vi "Areotech set reset.vi"(8 "error in (no error)":errorcluster, 10 "Parsed CMD":T1, 11 "AerotechStage in":refnum<class "AerotechStage.lvclass">) -> (0 "error out":errorcluster, 2 "new commands":string, 3 "AerotechStage out":refnum<class "AerotechStage.lvclass">)   [LabVIEW 2020, in "AerotechStage.lvclass"]
uses:
  AerotechStage.lvclass
  parsed device cmd.ctl
  OnOffTypeDef.ctl
  AerotechStage.lvclass/AerotechStage.ctl
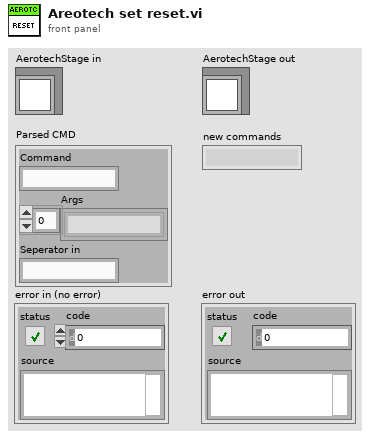
[diagram p1: front panel]
types:
  T1 = typedef "parsed device cmd.ctl" = cluster{"Command":string, "Args":string[], "Seperator in":string}
  T2 = typedef "OnOffTypeDef.ctl" = enum16{"off", "on"}
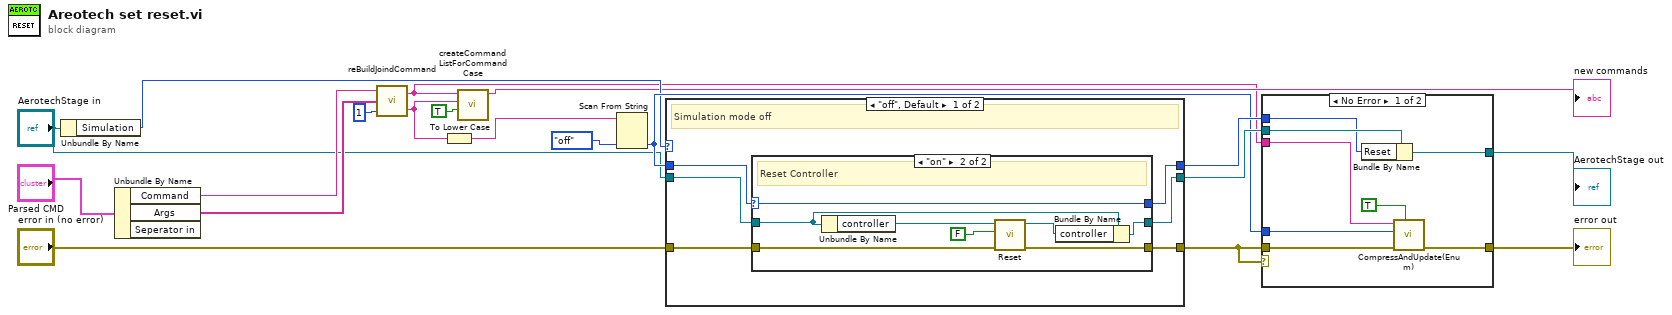
[diagram p0: block diagram]
diagram:
  n1 = Unbundle By Name("AerotechStage in") -> ("Simulation"=w7:T2)
  n2 = Unbundle By Name("Parsed CMD") -> ("Command"=w18:string, "Args"=w19:string[])  [unwired: 1 out]
  n3 = call "reBuildJoindCommand.vi"("number of group elements (0)"=1, "Args"=w19, "Command 2"=w18) -> ("Arg"=w9:string, "Command"=w3:string)
  n4 = To Lower Case(string=w9) -> (all lower case string=w8:string)
  n5 = call "createCommandListForCommandCase.vi"("immediate Check (only once)"=TRUE, "setvalue"=w9, "command"=w3) -> ("new commands"=→"new commands":string)  [unwired: 8 in]
  n6 = Scan From String(input string=w8, default 1=OnOffTypeDef."off" ("Settings.Enable.Axis 1")) -> (output 1=w11:T2)  [unwired: 3 in, 3 out]
  n7 = case shown="\"off\", Default" w7 {
    tunnel: "AerotechStage in" -> [w25 w39]
    tunnel: "error in (no error)" -> [w23 w38]
    tunnel: [w22 w38] -> w16
    tunnel: [w24 w39] -> w13
    tunnel: w11 -> [w21 w37]
    tunnel: [w20 w37] -> w15
    frame "off", Default {
      # "Simulation mode off"
      n8 = case shown="\"on\"" w21 {
        selector: w21 -> [w26 w29]
        tunnel: w25 -> [w27 w34]
        tunnel: [w27 w33] -> w24
        tunnel: w23 -> [w28 w36]
        tunnel: [w28 w35] -> w22
        tunnel: [w26 w29] -> w20
        frame "off", Default {
        }
        frame "on" {
          # "Reset Controller"
          n9 = Unbundle By Name(w34) -> ("controller"=w32:refnum<k24>)
          n10 = call "Reset.vi"("error in (no error)"=w36, "restart programs? (false)"=FALSE, "controller in"=w32) -> ("error out"=w35:errorcluster, "controller out"=w31:refnum<k24>)  [unwired: 7 in]
          n11 = Bundle By Name(cluster=w34, "controller"=w31) -> (w33:refnum<class "AerotechStage.lvclass">)
        }
      }
    }
    frame "on" {
      # "Simulation mode on"
    }
  }
  n12 = case shown="No Error" w16 {
    tunnel: w3 -> [w46 _]
    tunnel: w16 -> [w45 w49]
    tunnel: [w44 w49] -> w5
    tunnel: w11 -> [w43 _]
    tunnel: w13 -> [w42 w48]
    tunnel: [w41 w48] -> w14
    tunnel: w15 -> [w40 _]
    frame No Error {
      n13 = Bundle By Name(cluster=w42, "Reset"=w40) -> (w41:refnum<class "AerotechStage.lvclass">)
      n14 = call "CompressAndUpdate(Enum).vi"("force CVT update (false)"=TRUE, "error in"=w45, "enum variant"=w43, "command or variable name"=w46) -> ("error out"=w44:errorcluster)  [unwired: 7 in]
    }
    frame Error {
    }
  }
  "AerotechStage out" <- w14
  "error out" <- w5
